vi "Test New Node - UA Tree.vi"(8 "Error In":errorcluster, 11 "Server Connection Information":T1) -> (0 "Error Out":errorcluster)   [LabVIEW 2017, in "Unit Tests.lvlib"]
uses:
  Unit Tests.lvlib
  source/Browser Core/Server Classes/UA Server/Server Connection Information.ctl
  source/Browser Core/Node Classes/UA Node/UA Node.lvclass
  C:/Users/MattJ/Desktop/GitHubSCM/UA-Server-Browser/source/Browser Core/Node Classes/Generic Node/Generic Node.lvclass
  source/Browser Core/Node Classes/UA Node/Node Class.ctl
  source/Browser Core/Node Classes/Generic Node/Generic Node.lvclass/Generic Node.ctl
  source/Browser Core/Node Classes/UA Node/UA Node.lvclass/UA Node.ctl
  source/Browser Core/Server Classes/UA Server/UA Server.lvclass
  <vilib>/addons/_JKI Toolkits/Caraya/classes/Test/Test.lvclass
  source/Browser Core/Node Classes/Generic Node/Generic Node.lvclass
  <vilib>/addons/_JKI Toolkits/Caraya/classes/Assert/Assert.lvclass
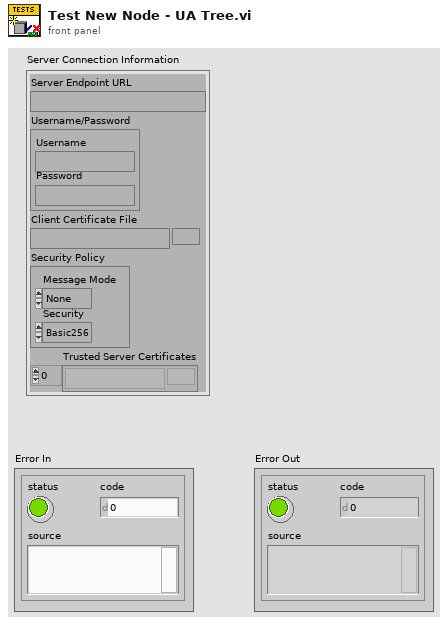
[diagram p1: front panel]
types:
  T1 = typedef "Browser Core.lvlib/UA Server.lvclass/Server Connection Information.ctl" = cluster{"Server Endpoint URL":string, "Username/Password":cluster{"Username":string, "Password":string}, "Client Certificate File":path, "Security Policy":cluster{"Message Mode":enum16{"None", "Sign", "Sign and Encrypt"}, "Security":enum16{"Basic256", "Basic128Rsa15"}}, "Trusted Server Certificates":path[]}
  T2 = typedef "Browser Core.lvlib/UA Node.lvclass/Node Class.ctl" = u16
  T3 = cluster{"Message Mode":enum16{"None", "Sign", "Sign and Encrypt"}, "Security":enum16{"Basic256", "Basic128Rsa15"}}
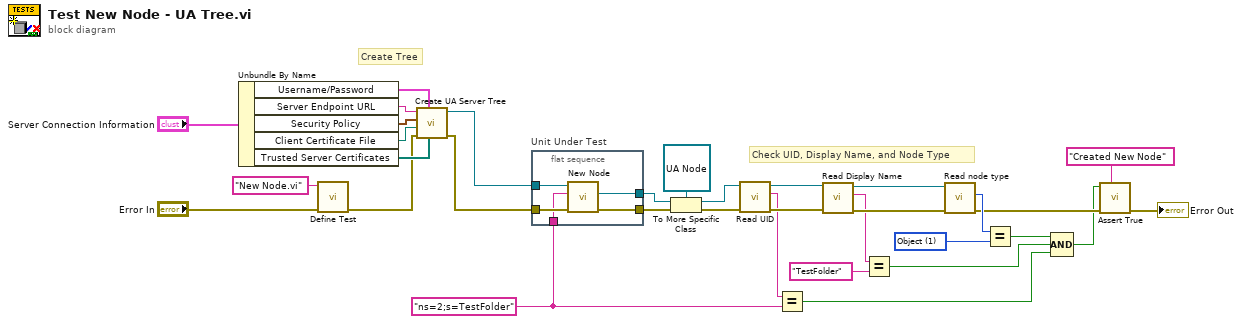
[diagram p0: block diagram]
diagram:
  w1 = T2 1 items=["Unspecified"=0, "Object"=1, "Variable"=2, "Method"=4, "Object Type"=8, "Variable Type"=16, "Reference Type"=32, "Data Type"=64, "View"=128] ("node class")
  w12 = "ns=2;s=TestFolder"
  # "Check UID, Display Name, and Node Type"
  # "Create Tree"
  n1 = Unbundle By Name("Server Connection Information") -> ("Username/Password"=w31:cluster{"Username":string, "Password":string}, "Server Endpoint URL"=w30:string, "Security Policy"=w29:T3, "Client Certificate File"=w28:path, "Trusted Server Certificates"=w27:path[])
  n2 = call <vilib>:"Define Test.vi"("error in (no error)"="Error In", "Label (VI Title)"="New Node.vi") -> ("error out"=w25:errorcluster)  [unwired: 9 in]
  n3 = call "Create UA Server Tree.vi"("Trusted Server Certificates"=w27, "Username/Password"=w31, "Error In"=w25, "Client Certificate File"=w28, "Security Policy"=w29, "Server Endpoint URL"=w30) -> ("Error Out"=w24:errorcluster, "UA Server Tree"=w23:refnum<class "UA Server.lvclass">)  [unwired: 4 in]
  n4 = flat-sequence "Unit Under Test" {
    tunnel: w23 -> [w38]
    tunnel: w24 -> [w37]
    tunnel: [w36] -> w22
    tunnel: [w35] -> w16
    tunnel: w12 -> [w34]
    frame #0 {
      n5 = call-dynamic "New Node.vi"("error in (no error)"=w37, "UID"=w34, "UA Server in"=w38) -> ("error out"=w35:errorcluster, "Generic Node out"=w36:refnum<class "Generic Node.lvclass">)  [unwired: 6 in, 1 out]
    }
  }
  n6 = To More Specific Class(target class=refnum<class "UA Node.lvclass"> refnum ("Browser Core.lvlib:UA Node.lvclass"), reference=w22, error in=w16) -> (specific class reference=w17:refnum<class "UA Node.lvclass">, error out=w15:errorcluster)
  n7 = call "Read UID.vi"("error in (no error)"=w15, "Generic Node in"=w17) -> ("error out"=w21:errorcluster, "UID"=w13:string, "Generic Node out"=w20:refnum<class "UA Node.lvclass">)  [unwired: 7 in]
  n8 = Equal?(x=w13, y=w12) -> (x = y?=w5:bool)
  n9 = call "Read Display Name.vi"("error in (no error)"=w21, "Generic Node in"=w20) -> ("error out"=w19:errorcluster, "Display Name"=w11:string, "Generic Node out"=w18:refnum<class "UA Node.lvclass">)  [unwired: 7 in]
  n10 = Equal?(x=w11, y="TestFolder") -> (x = y?=w6:bool)
  n11 = call "Read node type.vi"("error in (no error)"=w19, "UA Node in"=w18) -> ("error out"=w8:errorcluster, "node class"=w9:T2)  [unwired: 7 in, 1 out]
  n12 = Equal?(x=w9, y=w1) -> (x = y?=w7:bool)
  n13 = Compound Arithmetic op=AND(w7, w6, w5) -> (w4:bool)
  n14 = call <vilib>:"Assert True.vi"("Label"="Created New Node", "error in (no error)"=w8, "True?"=w4) -> ("error out"=→"Error Out":errorcluster)  [unwired: 8 in]
